vi "2023 Check for End Condition of FSM.vi"(2 "error in":errorcluster, 3 "armSensorPosition":dbl, 4 "wristSensorPosition":dbl) -> (0 "error out":errorcluster, 1 "timeToTransition":i32)   [LabVIEW 2020]
uses:
  2023 Robot Global Data.vi
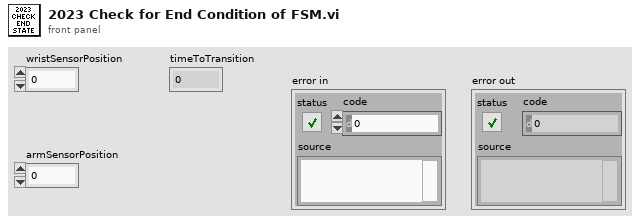
[diagram p1: front panel]
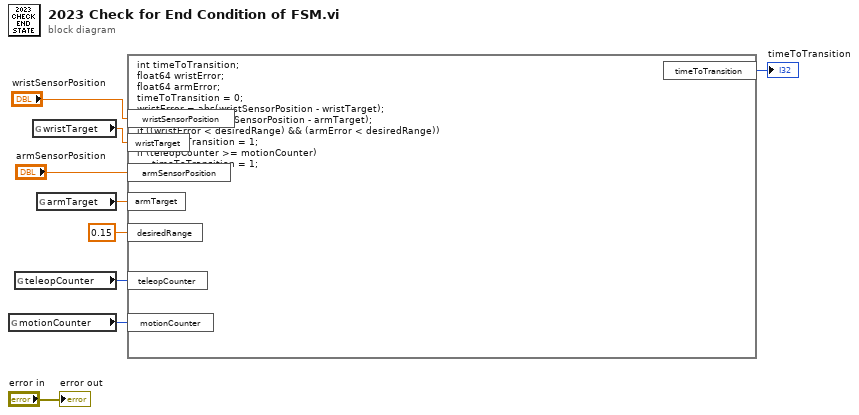
[diagram p0: block diagram]
diagram:
  n1 = global read "2023 Robot Global Data.vi" "motionCounter"() -> (w3:i32)
  n2 = global read "2023 Robot Global Data.vi" "teleopCounter"() -> (w9:i32)
  n3 = global read "2023 Robot Global Data.vi" "wristTarget"() -> (w7:dbl)
  n4 = global read "2023 Robot Global Data.vi" "armTarget"() -> (w8:dbl)
  n5 = formula code="int timeToTransition;\nfloat64 wristError;\nfloat64 armError;\ntimeToTransition = 0;\nwristError = abs(wristSensorPosition - wristTarget);\narmError = abs(armSensorPosition - armTarget);\nif ((wristError < desiredRange) && (armError < desiredRange))\n     timeToTransition = 1;\nif (teleopCounter >= motionCounter)\n     timeToTransition = 1;"("wristSensorPosition"="wristSensorPosition", "wristTarget"=w7, "armSensorPosition"="armSensorPosition", "armTarget"=w8, "teleopCounter"=w9, "motionCounter"=w3, "desiredRange"=0.15 ("input variable")) -> ("timeToTransition"=→"timeToTransition":i32)
  "error out" <- "error in"
